vi "Response TimeCalc.vi"(8 "dt (s)":dbl=2.0, 9 "Response":dbl[](array[numeric]), 10 "Setpoint":dbl) -> (2 "Response Time (s)":dbl)   [LabVIEW 2011]
doc: "This VI calculates whether a response acheived the specified <b>Response Time (s)</b>. It will also output the <b>Response Time (s)</b> for the value to go from the starting point to 70% of the value of the <b>Setpoint</b>."
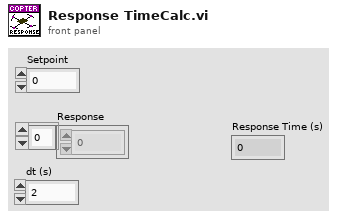
[diagram p1: front panel]
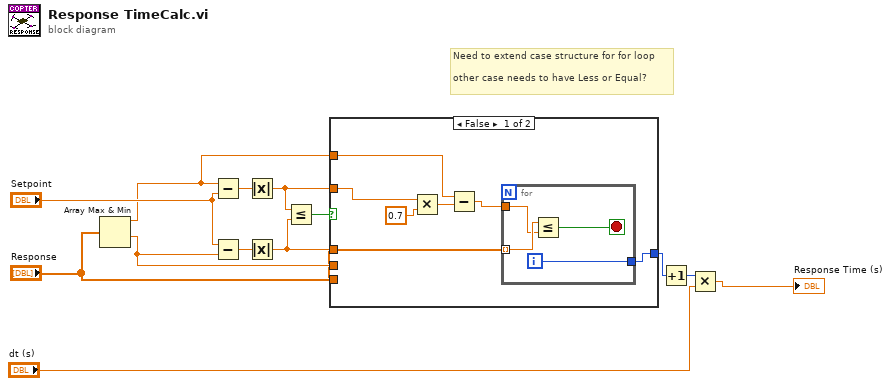
[diagram p0: block diagram]
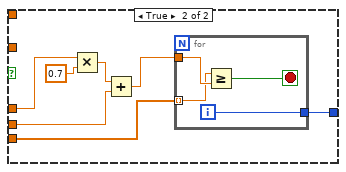
[diagram p2: hidden frame]
diagram:
  # "Need to extend case structure for for loop\n\nother case needs to have Less or Equal?"
  n1 = Array Max & Min(array="Response") -> (max value=w6:dbl, min value=w7:dbl)  [unwired: 2 out]
  n2 = Subtract(x=w6, y="Setpoint") -> (x-y=w10:dbl)
  n3 = Subtract(x="Setpoint", y=w7) -> (x-y=w11:dbl)
  n4 = Absolute Value(x=w10) -> (abs(x)=w5:dbl)
  n5 = Absolute Value(x=w11) -> (abs(x)=w8:dbl)
  n6 = Less Or Equal?(x=w5, y=w8) -> (x <= y?=w3:bool)
  n7 = case shown="False" w3 {
    tunnel: [w15 w31] -> w12
    tunnel: w8 -> [_ w29]
    tunnel: w7 -> [_ w28]
    tunnel: w6 -> [w18 _]
    tunnel: w5 -> [w14 _]
    tunnel: "Response" -> [w17 w25]
    frame False {
      n8 = Multiply(x=w14, y=0.7) -> (x*y=w20:dbl)
      n9 = Subtract(x=w18, y=w20) -> (x-y=w16:dbl)
      n10 = for {
        tunnel: [w23] -> w15
        tunnel: w17 -> [w22] mode=indexing
        tunnel: w16 -> [w21]
        i -> [w23]
        stop <- w24 stop-if-true
        n11 = Less Or Equal?(x=w22, y=w21) -> (x <= y?=w24:bool)
      }
    }
    frame True {
      n12 = Multiply(x=w29, y=0.7) -> (x*y=w26:dbl)
      n13 = Add(x=w26, y=w28) -> (x+y=w30:dbl)
      n14 = for {
        tunnel: w30 -> [w34]
        tunnel: [w33] -> w31
        tunnel: w25 -> [w32] mode=indexing
        i -> [w33]
        stop <- w35 stop-if-true
        n15 = Greater Or Equal?(x=w32, y=w34) -> (x >= y?=w35:bool)
      }
    }
  }
  n16 = Increment(x=w12) -> (x+1=w13:i32)
  n17 = Multiply(x=w13, y="dt (s)") -> (x*y=→"Response Time (s)":dbl)
